vi "Inline - Update Status Channels - Get Index and Value from Channel Name.vi"(9 "Time (us)/Error Counter Value":u32, 10 "Error Code":i32, 11 "Status Channel":T1) -> (2 "Value":dbl, 3 "index":i32)   [LabVIEW 2020, in "Ballard Arinc-429 Engine.lvlib"]
uses:
  Ballard Arinc-429 Engine.lvlib
  RT Controls/Inline_Status_Channels.ctl
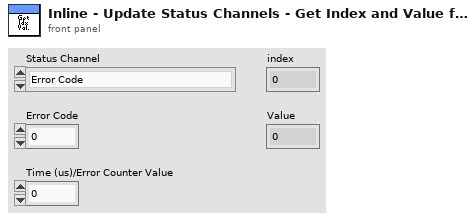
[diagram p1: front panel]
types:
  T1 = typedef "Ballard Arinc-429 Engine.lvlib/Inline_Status_Channels.ctl" = enum16{"Error Code", "Inline Read Time (us)", "Inline Write Time (us)", "Receiving Error - Error Counter", "Gap Error - Error Counter", "Parity Error - Error Counter", "Long Word Error - Error Counter", "Bit Timing Error - Error Counter"}
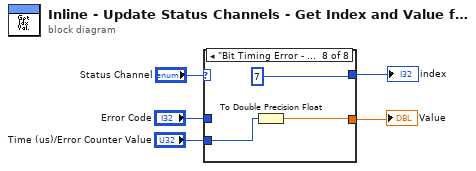
[diagram p0: block diagram]
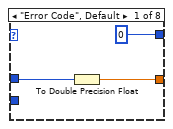
[diagram p2: hidden frame]
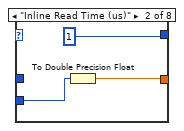
[diagram p3: hidden frame]
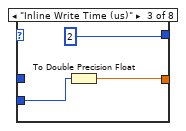
[diagram p4: hidden frame]
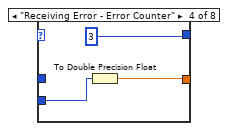
[diagram p5: hidden frame]
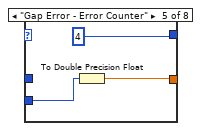
[diagram p6: hidden frame]
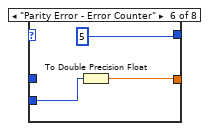
[diagram p7: hidden frame]
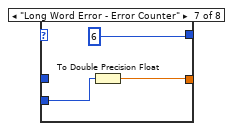
[diagram p8: hidden frame]
diagram:
  n1 = case shown="\"Bit Timing Error - Error Counter\"" "Status Channel" {
    tunnel: [0 ("index") 1 ("index") 2 ("index") 3 ("index") 4 ("index") 5 ("index") 6 ("index") 7 ("index")] -> w1
    tunnel: "Error Code" -> [w7 _ _ _ _ _ _ _]
    tunnel: [w6 w10 w13 w16 w19 w22 w25 w28] -> w4
    tunnel: "Time (us)/Error Counter Value" -> [_ w9 w12 w15 w18 w21 w24 w27]
    frame "Error Code", Default {
      n2 = To Double Precision Float(number=w7) -> (double precision float=w6:dbl)
    }
    frame "Inline Read Time (us)" {
      n3 = To Double Precision Float(number=w9) -> (double precision float=w10:dbl)
    }
    frame "Inline Write Time (us)" {
      n4 = To Double Precision Float(number=w12) -> (double precision float=w13:dbl)
    }
    frame "Receiving Error - Error Counter" {
      n5 = To Double Precision Float(number=w15) -> (double precision float=w16:dbl)
    }
    frame "Gap Error - Error Counter" {
      n6 = To Double Precision Float(number=w18) -> (double precision float=w19:dbl)
    }
    frame "Parity Error - Error Counter" {
      n7 = To Double Precision Float(number=w21) -> (double precision float=w22:dbl)
    }
    frame "Long Word Error - Error Counter" {
      n8 = To Double Precision Float(number=w24) -> (double precision float=w25:dbl)
    }
    frame "Bit Timing Error - Error Counter" {
      n9 = To Double Precision Float(number=w27) -> (double precision float=w28:dbl)
    }
  }
  "Value" <- w4
  "index" <- w1
